vi "AB_User_Log_FileIO.vi"(6 "file":path, 7 "fileAction":T1, 8 "error in (no error)":errorcluster, 10 "data":string, 11 "newSection":string) -> (0 "error out":errorcluster)   [LabVIEW 2020]
uses:
  <vilib>/AppBuilder/logging/AB_Log_File_Action.ctl
  <resource>/Framework/Providers/Common/provcom_StringGlobals.vi
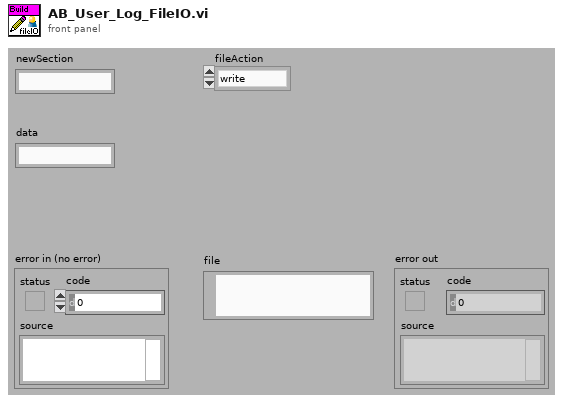
[diagram p1: front panel]
types:
  T1 = typedef "AB_Log_File_Action.ctl" = enum16{"write", "open", "close"}
  T2 = enum16{"open", "open or create", "create or replace", "create", "open (read only)"}
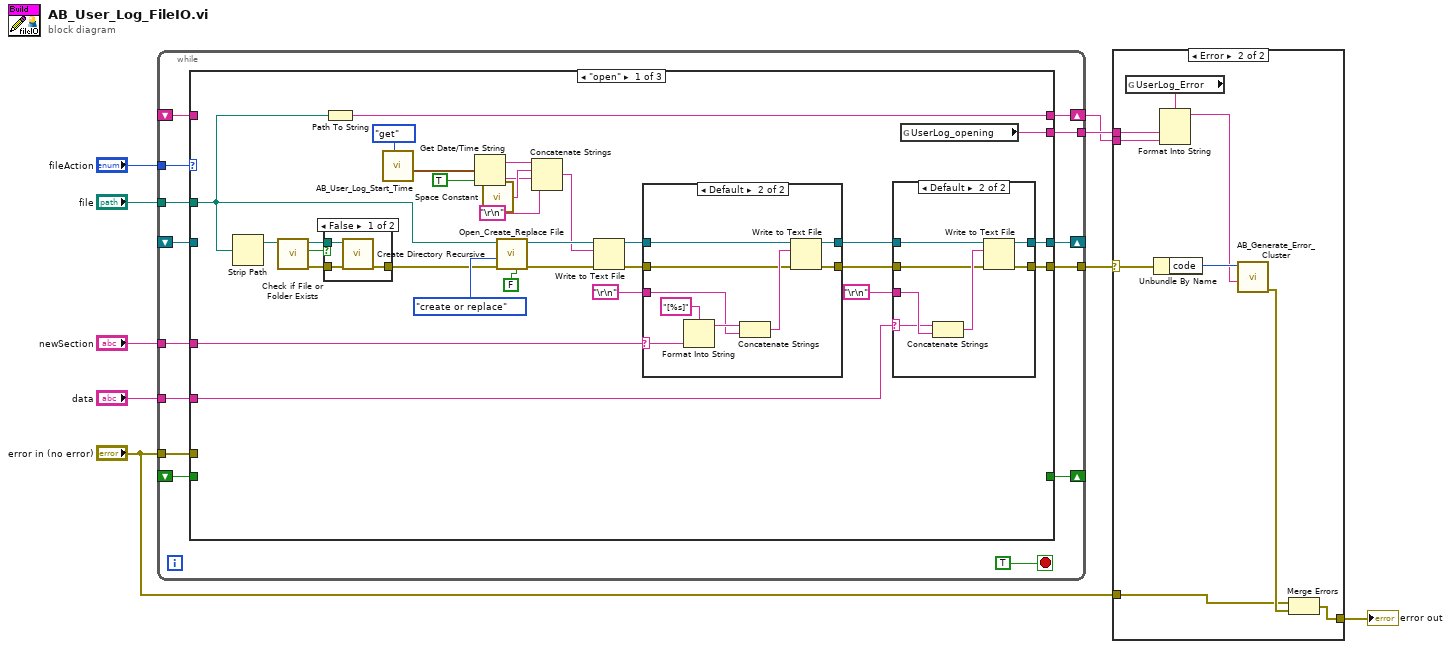
[diagram p0: block diagram]
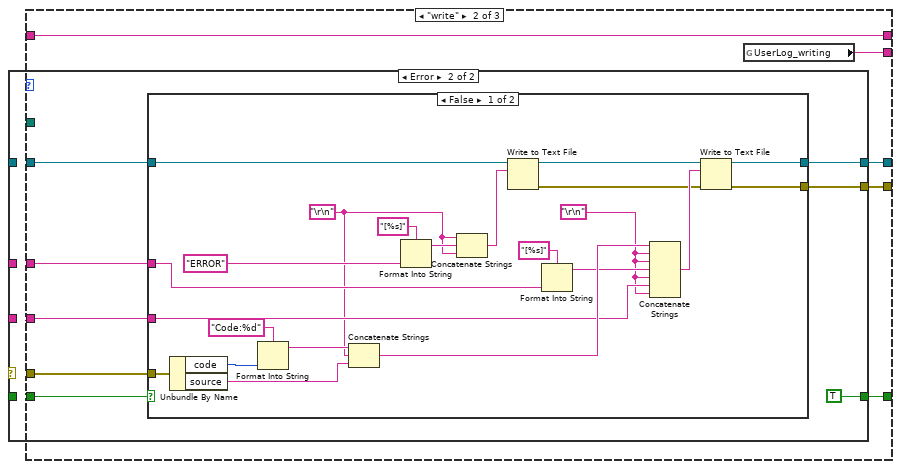
[diagram p6: hidden frame]
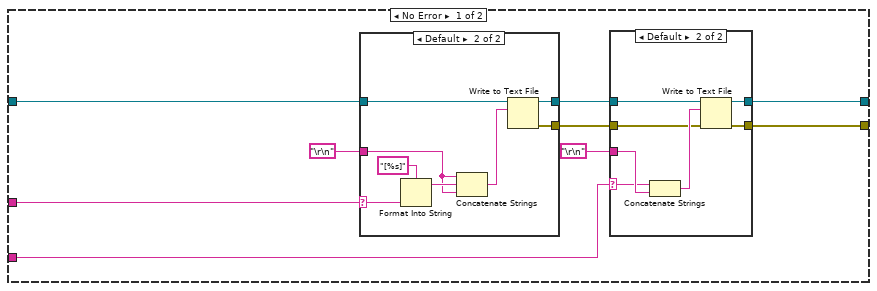
[diagram p7: hidden frame]
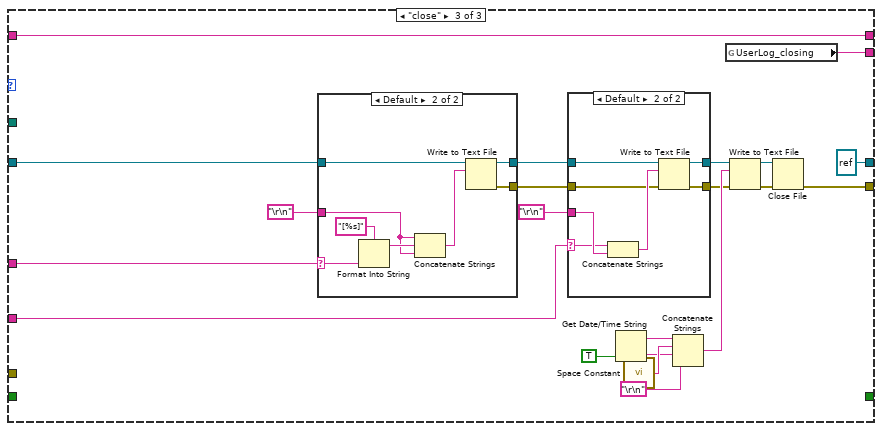
[diagram p11: hidden frame]
diagram:
  n1 = while {
    tunnel: "fileAction" -> [w22]
    tunnel: "file" -> [w21]
    shift-right: [w20] -> _
    shift-left: _ -> [w17]
    tunnel: "newSection" -> [w19]
    tunnel: "data" -> [w18]
    tunnel: "error in (no error)" -> [w16]
    shift-right: [w15] -> _
    shift-left: _ -> [w14]
    tunnel: [w13] -> w3
    shift-right: [w12] -> w4
    shift-left: _ -> [w11]
    tunnel: [w10] -> w5
    stop <- TRUE stop-if-true
    n2 = case shown="\"open\"" w22 {
      tunnel: w21 -> [w24 _ _]
      tunnel: [w53 w87 refnum<file> refnum ("refnum out")] -> w20
      tunnel: w19 -> [w51 w84 w164]
      tunnel: w18 -> [w52 w86 w166]
      tunnel: w17 -> [_ w85 w165]
      tunnel: w16 -> [_ w83 _]
      tunnel: [_ w82 _] -> w15
      tunnel: w14 -> [_ w81 _]
      tunnel: [w32 w80 w148] -> w13
      tunnel: [w31 w79 w147] -> w12
      tunnel: w11 -> [_ w79 w147]
      tunnel: [w30 w78 w146] -> w10
      frame "open" {
        n3 = Strip Path(path=w24) -> (stripped path=w29:path)  [unwired: 1 out]
        n4 = call <vilib>:"Check if File or Folder Exists.vi"("path"=w29) -> ("error out"=w27:errorcluster, "file or folder exists?"=w28:bool, "dup path"=w26:path)  [unwired: 8 in]
        n5 = case shown="False" w28 {
          tunnel: w27 -> [w56 w57]
          tunnel: [w55 w57] -> w25
          tunnel: w26 -> [w54 _]
          frame False {
            n6 = call <vilib>:"Create Directory Recursive.vi"("error in (no error)"=w56, "directory"=w54) -> ("error out"=w55:errorcluster)  [unwired: 3 in, 2 out]
          }
          frame True {
          }
        }
        n7 = Path To String(path=w24) -> (string=w31:string)
        n8 = call <vilib>:"AB_User_Log_Start_Time.vi"("action"=enum16{"get", "set"}."get") -> ("start time"=w36:timestamp)  [unwired: 1 in, 9 out]
        n9 = Get Date/Time String(seconds (now)=w36, want seconds? (F)=TRUE) -> (date string=w42:string, time string=w40:string)  [unwired: 1 in]
        n10 = call <vilib>:"Space Constant.vi"() -> ("String"=w41:string)
        n11 = call <vilib>:"Open_Create_Replace File.vi"("advisory dialog? (display:T)"=FALSE, "error in (no error)"=w25, "function (open:0)"=T2."create or replace", "file path"=w24) -> ("error out"=w35:errorcluster, "refnum"=w45:refnum<file>)  [unwired: 3 in, 3 out]
        n12 = Concatenate Strings(w42, w41, w40, "\r\n") -> (w38:string)
        n13 = Write to Text File(file (use dialog)=w45, text=w38, error in=w35) -> (refnum out=w44:refnum<file>, error out=w34:errorcluster)  [unwired: 2 out]
        n14 = case shown="Default" w51 {
          selector: w51 -> [_ w73]
          tunnel: w44 -> [w68 w77]
          tunnel: [w68 w76] -> w48
          tunnel: "\r\n" -> [_ w71]
          tunnel: w34 -> [w67 w70]
          tunnel: [w67 w69] -> w33
          frame "" {
          }
          frame Default {
            n15 = Format Into String(format string="[%s]", w73) -> (resulting string=w72:string)  [unwired: 2 in, 1 out]
            n16 = Concatenate Strings(w72, w71) -> (w75:string)
            n17 = Write to Text File(file (use dialog)=w77, text=w75, error in=w70) -> (refnum out=w76:refnum<file>, error out=w69:errorcluster)  [unwired: 2 out]
          }
        }
        n18 = case shown="Default" w52 {
          selector: w52 -> [_ w62]
          tunnel: w48 -> [w59 w66]
          tunnel: [w59 w65] -> w53
          tunnel: "\r\n" -> [_ w63]
          tunnel: w33 -> [w58 w61]
          tunnel: [w58 w60] -> w32
          frame "" {
          }
          frame Default {
            n19 = Concatenate Strings(w62, w63) -> (w64:string)
            n20 = Write to Text File(file (use dialog)=w66, text=w64, error in=w61) -> (refnum out=w65:refnum<file>, error out=w60:errorcluster)  [unwired: 2 out]
          }
        }
        n21 = global read "provcom_StringGlobals.vi" "UserLog_opening"() -> (w30:string)
      }
      frame "write" {
        n22 = case shown="Error" w83 {
          selector: w83 -> [_ w116]
          tunnel: [w90 w119] -> w87
          tunnel: w86 -> [w93 w120]
          tunnel: w85 -> [w96 w122]
          tunnel: w84 -> [w95 w121]
          tunnel: [_ TRUE] -> w82
          tunnel: w81 -> [_ w117]
          tunnel: [w88 w115] -> w80
          frame No Error {
            n23 = case shown="Default" w95 {
              selector: w95 -> [_ w110]
              tunnel: w96 -> [w106 w114]
              tunnel: [w106 w113] -> w91
              tunnel: "\r\n" -> [_ w108]
              tunnel: [_ w107] -> w89
              frame "" {
              }
              frame Default {
                n24 = Format Into String(format string="[%s]", w110) -> (resulting string=w109:string)  [unwired: 2 in, 1 out]
                n25 = Concatenate Strings(w108, w109, w108) -> (w112:string)
                n26 = Write to Text File(file (use dialog)=w114, text=w112) -> (refnum out=w113:refnum<file>, error out=w107:errorcluster)  [unwired: 1 in, 2 out]
              }
            }
            n27 = case shown="Default" w93 {
              selector: w93 -> [_ w101]
              tunnel: w91 -> [w98 w105]
              tunnel: [w98 w104] -> w90
              tunnel: "\r\n" -> [_ w102]
              tunnel: w89 -> [w97 w100]
              tunnel: [w97 w99] -> w88
              frame "" {
              }
              frame Default {
                n28 = Concatenate Strings(w101, w102) -> (w103:string)
                n29 = Write to Text File(file (use dialog)=w105, text=w103, error in=w100) -> (refnum out=w104:refnum<file>, error out=w99:errorcluster)  [unwired: 2 out]
              }
            }
          }
          frame Error {
            n30 = case shown="False" w117 {
              tunnel: w122 -> [w144 w145]
              tunnel: w121 -> [w128 _]
              tunnel: w120 -> [w130 _]
              tunnel: [w142 w145] -> w119
              tunnel: w116 -> [w141 _]
              tunnel: [w123 _] -> w115
              frame False {
                w126 = "\r\n"
                w125 = "\r\n"
                n31 = Unbundle By Name(w141) -> ("code"=w138:i32, "source"=w136:string)
                n32 = Format Into String(format string="Code:%d", w138) -> (resulting string=w137:string)  [unwired: 2 in, 1 out]
                n33 = Concatenate Strings(w137, w125, w136) -> (w135:string)
                n34 = Format Into String(format string="[%s]", "ERROR" ("format string")) -> (resulting string=w131:string)  [unwired: 2 in, 1 out]
                n35 = Concatenate Strings(w125, w131, w125) -> (w133:string)
                n36 = Write to Text File(file (use dialog)=w144, text=w133) -> (refnum out=w143:refnum<file>, error out=w124:errorcluster)  [unwired: 1 in, 2 out]
                n37 = Format Into String(format string="[%s]", w128) -> (resulting string=w127:string)  [unwired: 2 in, 1 out]
                n38 = Concatenate Strings(w135, w126, w126, w127, w126, w130, w126) -> (w134:string)
                n39 = Write to Text File(file (use dialog)=w143, text=w134, error in=w124) -> (refnum out=w142:refnum<file>, error out=w123:errorcluster)  [unwired: 2 out]
              }
              frame True {
              }
            }
          }
        }
        n40 = global read "provcom_StringGlobals.vi" "UserLog_writing"() -> (w78:string)
      }
      frame "close" {
        n41 = case shown="Default" w164 {
          selector: w164 -> [_ w179]
          tunnel: w165 -> [w175 w183]
          tunnel: [w175 w182] -> w161
          tunnel: "\r\n" -> [_ w177]
          tunnel: [_ w176] -> w151
          frame "" {
          }
          frame Default {
            n42 = Format Into String(format string="[%s]", w179) -> (resulting string=w178:string)  [unwired: 2 in, 1 out]
            n43 = Concatenate Strings(w177, w178, w177) -> (w181:string)
            n44 = Write to Text File(file (use dialog)=w183, text=w181) -> (refnum out=w182:refnum<file>, error out=w176:errorcluster)  [unwired: 1 in, 2 out]
          }
        }
        n45 = case shown="Default" w166 {
          selector: w166 -> [_ w170]
          tunnel: w161 -> [w167 w174]
          tunnel: [w167 w173] -> w155
          tunnel: "\r\n" -> [_ w171]
          tunnel: w151 -> [_ w169]
          tunnel: [_ w168] -> w150
          frame "" {
          }
          frame Default {
            n46 = Concatenate Strings(w170, w171) -> (w172:string)
            n47 = Write to Text File(file (use dialog)=w174, text=w172, error in=w169) -> (refnum out=w173:refnum<file>, error out=w168:errorcluster)  [unwired: 2 out]
          }
        }
        n48 = Get Date/Time String(want seconds? (F)=TRUE) -> (date string=w159:string, time string=w157:string)  [unwired: 2 out]
        n49 = call <vilib>:"Space Constant.vi"() -> ("String"=w158:string)
        n50 = Concatenate Strings(w159, w158, w157, "\r\n") -> (w153:string)
        n51 = global read "provcom_StringGlobals.vi" "UserLog_closing"() -> (w146:string)
        n52 = Write to Text File(file (use dialog)=w155, text=w153, error in=w150) -> (refnum out=w154:refnum<file>, error out=w149:errorcluster)  [unwired: 2 out]
        n53 = Close File(refnum=w154, error in=w149) -> (error out=w148:errorcluster)  [unwired: 1 out]
      }
    }
  }
  n54 = case shown="Error" w3 {
    selector: w3 -> [_ w188]
    tunnel: w5 -> [_ w190]
    tunnel: w4 -> [_ w189]
    tunnel: "error in (no error)" -> [w184 w186]
    tunnel: [w184 w185] -> w1
    frame No Error {
    }
    frame Error {
      n55 = global read "provcom_StringGlobals.vi" "UserLog_Error"() -> (w192:string)
      n56 = Unbundle By Name(w188) -> ("code"=w193:i32)
      n57 = Format Into String(format string=w192, w190, w189) -> (resulting string=w191:string)  [unwired: 2 in, 1 out]
      n58 = call <vilib>:"AB_Generate_Error_Cluster.vi"("Additional Message"=w191, "Code"=w193) -> ("error out"=w187:errorcluster)  [unwired: 9 in]
      n59 = Merge Errors(w186, w187) -> (w185:errorcluster)
    }
  }
  "error out" <- w1
